vi "Discard Non-Analog Channels MUX80.vi"(7 "Channels In (-)":i32[](array[numeric])=[31, 31, 31, 31, 31, 31, 31, 31, 31, 31, 31, 31, 31, 31, 31, 31], 9 "Ranges In":string[](array[string]), 10 "Channels In":i32[](array[numeric])) -> (1 "Ranges Out":string[](array[string]), 2 "Channels Out":i32[](array[numeric]), 4 "FIO/EIO Analog Enable":i32, 5 "Channels Out (-)":i32[](array[numeric]))   [LabVIEW 2020]
panel:
  # "This is a simply VI to remove non-analog channels from the channels/ranges arrays.  The output\narrays contain analog channels only and can then be used to configure ranges.  Also calculates\nthe value to pass to enable the needed analog channels on the U3."
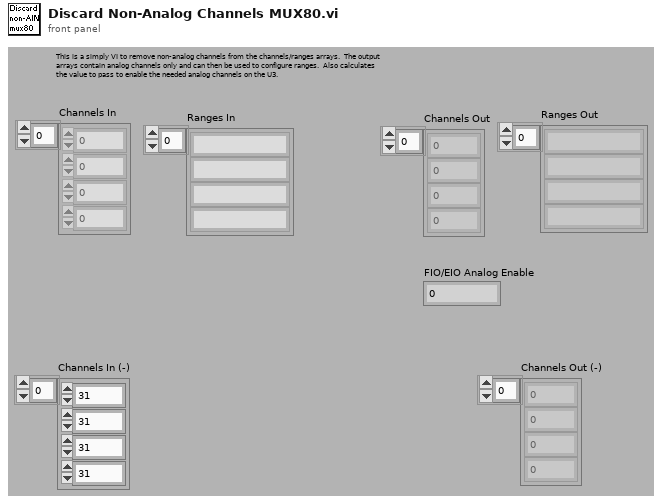
[diagram p1: front panel]
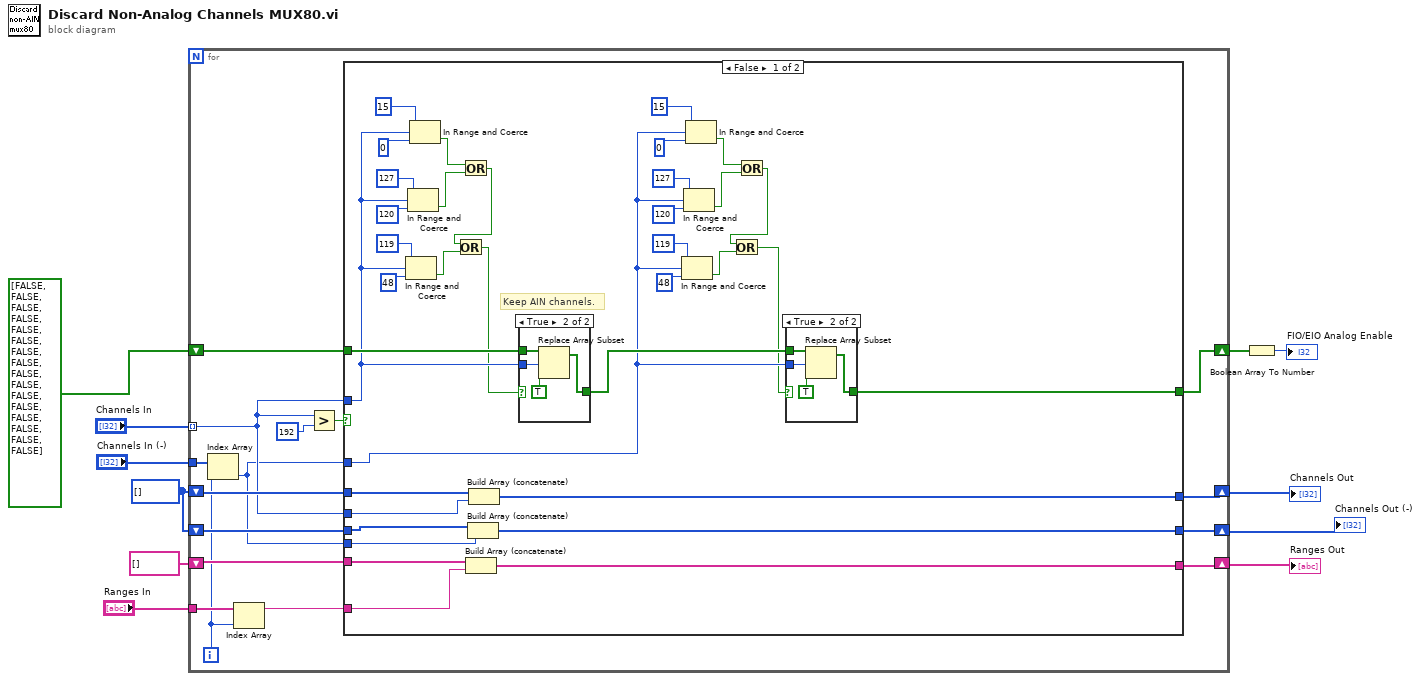
[diagram p0: block diagram]
diagram:
  w3 = i32[] []
  n1 = for {
    shift-right: [w25] -> w8
    shift-left: w3 -> [w26]
    shift-right: [w22] -> w7
    shift-left: string[] [] -> [w23]
    tunnel: "Channels In" -> [w21] mode=indexing
    tunnel: "Ranges In" -> [w18]
    shift-right: [w19] -> w5
    shift-left: bool[] [FALSE, FALSE, FALSE, FALSE, FALSE, FALSE, FALSE, FALSE, FALSE, FALSE, FALSE, FALSE, FALSE, FALSE, FALSE, FALSE] -> [w20]
    shift-right: [w16] -> w1
    shift-left: w3 -> [w15]
    tunnel: "Channels In (-)" -> [w14]
    i -> [w13]
    n2 = Index Array(array=w14, index=w13) -> (element=w12:i32)
    n3 = Index Array(array=w18, index=w13) -> (element=w17:string)
    n4 = Greater?(x=w21, y=192) -> (0:w27:bool)
    n5 = case shown="False" w27 {
      tunnel: w21 -> [w62 _]
      tunnel: w26 -> [w63 w77]
      tunnel: [w61 w77] -> w25
      tunnel: w23 -> [w60 w76]
      tunnel: w17 -> [w59 _]
      tunnel: [w58 w76] -> w22
      tunnel: w21 -> [w45 _]
      tunnel: w20 -> [w55 w75]
      tunnel: [w50 w75] -> w19
      tunnel: [w54 w74] -> w16
      tunnel: w15 -> [w52 w74]
      tunnel: w12 -> [w53 _]
      tunnel: w12 -> [w29 _]
      frame False {
        # "Keep AIN channels."
        n6 = In Range and Coerce(upper limit=119, x=w45, lower limit=48) -> (In Range?=w42:bool)  [unwired: 1 out]
        n7 = In Range and Coerce(upper limit=127, x=w45, lower limit=120) -> (In Range?=w43:bool)  [unwired: 1 out]
        n8 = In Range and Coerce(upper limit=15, x=w45, lower limit=0) -> (In Range?=w44:bool)  [unwired: 1 out]
        n9 = Or(x=w44, y=w43) -> (x .or. y?=w41:bool)
        n10 = Or(x=w41, y=w42) -> (x .or. y?=w40:bool)
        n11 = Build Array (concatenate)(w60, w59) -> (w58:string[])
        n12 = Build Array (concatenate)(w52, w53) -> (w54:i32[])
        n13 = Build Array (concatenate)(w63, w62) -> (w61:i32[])
        n14 = case shown="True" w40 {
          tunnel: w55 -> [w69 w72]
          tunnel: [w69 w70] -> w51
          tunnel: w45 -> [_ w73]
          frame False {
          }
          frame True {
            n15 = Replace Array Subset(array=w72, new element=TRUE, index=w73) -> (w70:bool[])
          }
        }
        n16 = In Range and Coerce(upper limit=119, x=w29, lower limit=48) -> (In Range?=w31:bool)  [unwired: 1 out]
        n17 = In Range and Coerce(upper limit=127, x=w29, lower limit=120) -> (In Range?=w32:bool)  [unwired: 1 out]
        n18 = In Range and Coerce(upper limit=15, x=w29, lower limit=0) -> (In Range?=w33:bool)  [unwired: 1 out]
        n19 = Or(x=w33, y=w32) -> (x .or. y?=w30:bool)
        n20 = Or(x=w30, y=w31) -> (x .or. y?=w28:bool)
        n21 = case shown="True" w28 {
          tunnel: w51 -> [w64 w67]
          tunnel: [w64 w65] -> w50
          tunnel: w29 -> [_ w68]
          frame False {
          }
          frame True {
            n22 = Replace Array Subset(array=w67, new element=TRUE, index=w68) -> (w65:bool[])
          }
        }
      }
      frame True {
      }
    }
  }
  "Channels Out" <- w8
  "Ranges Out" <- w7
  "Channels Out (-)" <- w1
  n23 = Boolean Array To Number(Boolean array=w5) -> (number=→"FIO/EIO Analog Enable":u32)
